vi "Plot xy Data and Print.vi"(0 "File:":string, 4 "Data":dbl[][](array[numeric]) format="%.2e", 5 "x axis column":i32, 6 "Column Headings":string[](array[string])=["Current", "Previous"], 7 "Display/hide":bool[](array[boolean]), 8 "X-Axis Data":dbl[][](array[numeric]) format="%.2e", 9 "Print":bool, 10 "Index":i32) -> (2 "x axis label":string, 3 "Data Plot":cluster{dbl[], dbl[]}[](graph))   [LabVIEW 2025]
doc: "Author: Scott Hannahs <sth@magnet.fsu.edu>\n\nThis software is licensed for use under the “MIT License\"\nCopyright (c) 2025 Scott Hannahs, sth@sth@magnet.sthnet.net\n\nPermission is hereby granted, free of charge, to any person obtaining a copy of this software and associated documentation files (the \"Software\"), to deal in the Software without restriction, including without limitation the rights to use, copy, modify, merge, publish, distribute, sublicense, and/or sell copies of the Software, and to permit persons to whom the Software is furnished to do so, subject to the following conditions: The above copyright notice and this permission notice shall be included in all copies or substantial portions of the Software.\n\nTHE SOFTWARE IS PROVIDED \"AS IS\", WITHOUT WARRANTY OF ANY KIND, EXPRESS OR IMPLIED, INCLUDING BUT NOT LIMITED TO THE WARRANTIES OF MERCHANTABILITY, FITNESS FOR A PARTICULAR PURPOSE AND NONINFRINGEMENT. IN NO EVENT SHALL THE AUTHORS OR COPYRIGHT HOLDERS BE LIABLE FOR ANY CLAIM, DAMAGES OR OTHER LIABILITY, WHETHER IN AN ACTION OF CONTRACT, TORT OR OTHERWISE, ARISING FROM, OUT OF OR IN CONNECTION WITH THE SOFTWARE OR THE USE OR OTHER DEALINGS IN THE SOFTWARE."
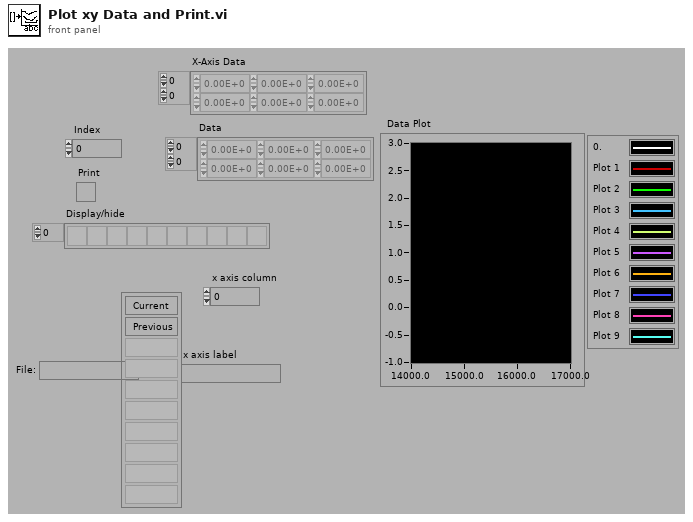
[diagram p1: front panel]
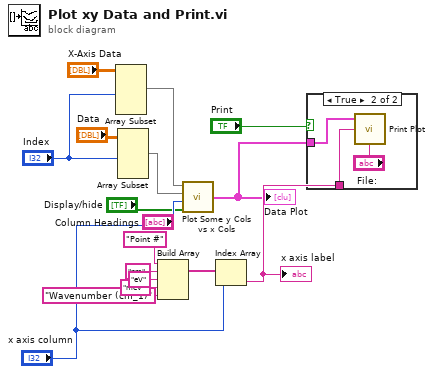
[diagram p0: block diagram]
diagram:
  n1 = Array Subset(array="X-Axis Data", length (row)="Index") -> (w5:dbl[][])  [unwired: 3 in]
  n2 = Array Subset(array="Data", length (row)="Index") -> (w11:dbl[][])  [unwired: 3 in]
  n3 = Build Array("Point #", "nm" ("Input Element"), "eV" ("Input Element"), "meV" ("Input Element"), "Wavenumber (cm_1)" ("Input Element")) -> (w15:string[])
  n4 = call "Plot Some y Cols vs x Cols.vi"("Display/hide"="Display/hide", "X-Axis Selection"="x axis column", "Input Array"=w11, "Input X-Axis Array"=w5) -> ("Output Graph"=w8:cluster{dbl[], dbl[]}[])
  "Data Plot" <- w8
  n5 = Index Array(array=w15, index="x axis column") -> (element=w14:string)
  "x axis label" <- w14
  n6 = case shown="True" "Print" {
    tunnel: w14 -> [_ w18]
    tunnel: w8 -> [_ w17]
    frame False {
    }
    frame True {
      n7 = call "Print Plot.vi"("File:"="File:", "X-Axis Label"=w18, "Data Plot"=w17) -> ()
    }
  }
